vi "SV Append Waveforms (N Ch) (DBL).vi"(7 "reset (F)":bool, 8 "error in (no error)":errorcluster, 10 "maximum length [s] (-1 = unlimited)":dbl=-1.0, 11 "waveform data in":waveform(dbl)[](array[waveform])) -> (0 "error out":errorcluster, 3 "appended waveform data":waveform(dbl)[](array[waveform]))   [LabVIEW 2017]
doc: "Use this VI to buffer data by appending input data to previously buffered data. Set the <B>maximum length</B> to set the buffered array size. The VI functions like a FIFO (First In, First Out) buffer, meaning that the oldest data is overwritten as new elements are added to the buffer. Wire data to the <B>data in</B> input to determine the polymorphic instance to use or manually select the instance."
uses:
  <vilib>/addons/_NISVFA/_Shared subVIs/Common/svc_Get Waveform Subset (Index).vi
  <vilib>/addons/_NISVFA/_Shared subVIs/Common/svc_Check for Waveform Parameter Continuity (no state).vi
  <vilib>/addons/_NISVFA/_Shared subVIs/Common/svc_Get Array Subset (Index).vi
  <vilib>/addons/_NISVFA/_Shared subVIs/Common/svc_Get SV Channel Info.vi
  <vilib>/addons/_NISVFA/_Shared subVIs/Common/svc_Coerce Index and Length.vi
  <vilib>/addons/_NISVFA/_Shared subVIs/Common/svc_Conditional Merge Error.vi
  <vilib>/addons/_NISVFA/_Shared subVIs/Common/svc_Engineering Units to Unit Label.vi
  <vilib>/addons/_NISVFA/_Shared subVIs/Common/svc_Unit Label to Engineering Units.vi
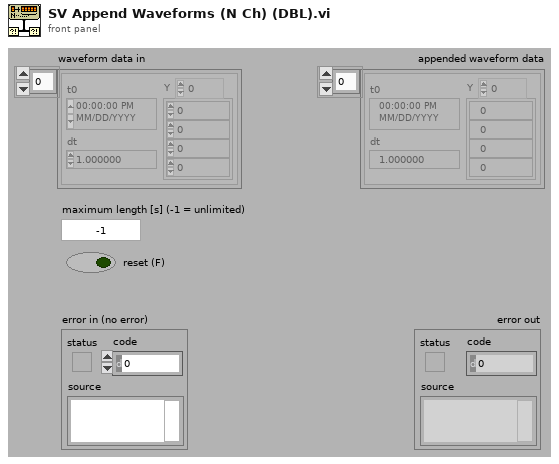
[diagram p1: front panel]
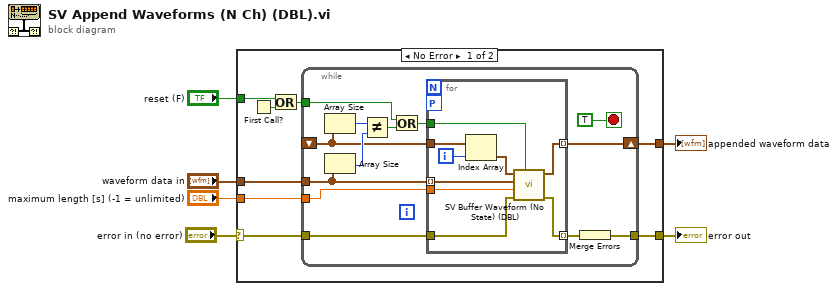
[diagram p0: block diagram]
diagram:
  n1 = case shown="No Error" "error in (no error)" {
    selector: "error in (no error)" -> [w7 w38]
    tunnel: "reset (F)" -> [w14 _]
    tunnel: [w12 w37] -> w5
    tunnel: "maximum length [s] (-1 = unlimited)" -> [w11 _]
    tunnel: "waveform data in" -> [w10 w37]
    tunnel: [w8 w38] -> w2
    frame No Error {
      n2 = First Call?() -> (First Call?: T/F=w9:bool)
      n3 = Or(x=w14, y=w9) -> (x .or. y?=w13:bool)
      n4 = while {
        tunnel: w10 -> [w24]
        shift-right: [w27] -> w12
        shift-left: _ -> [w18]
        tunnel: w11 -> [w25]
        tunnel: w13 -> [w20]
        tunnel: w7 -> [w17]
        tunnel: [w15] -> w8
        stop <- TRUE stop-if-true
        n5 = Array Size(array=w18) -> (size(s)=w23:i32)
        n6 = Array Size(array=w24) -> (size(s)=w22:i32)
        n7 = Not Equal?(x=w23, y=w22) -> (x != y?=w21:bool)
        n8 = Or(x=w20, y=w21) -> (x .or. y?=w19:bool)
        n9 = for {
          tunnel: [w36] -> w27 mode=indexing
          tunnel: w18 -> [w32]
          tunnel: w24 -> [w35] mode=indexing
          tunnel: w19 -> [w34]
          tunnel: w25 -> [w33]
          workers-P: _ -> [_]
          tunnel: w17 -> [w29]
          tunnel: [w28] -> w16 mode=indexing
          i -> [w30]
          n10 = Index Array(array=w32, index=w30) -> (element=w31:waveform(dbl))
          n11 = call <vilib>:"SV Buffer Waveform (No State) (DBL).vi"("clear buffer (False)"=w34, "error in (no error)"=w29, "buffer length [s] (-1 = unlimited)"=w33, "waveform"=w35, "buffer in"=w31) -> ("error out"=w28:errorcluster, "buffer out"=w36:waveform(dbl))  [unwired: 5 in]
        }
        n12 = Merge Errors(w16) -> (w15:errorcluster)
      }
    }
    frame Error {
    }
  }
  "appended waveform data" <- w5
  "error out" <- w2
